vi "AKD Set Drive Enable.vi"(0 "connection ID":refnum<k5>, 11 "error in":errorcluster) -> (4 "TCP Refnum":refnum<k5>, 15 "error out":errorcluster)   [LabVIEW 2019]
uses:
  MODBUS/NI Modbus.llb/MB Ethernet Master Query Write Multiple Registers (poly).vi
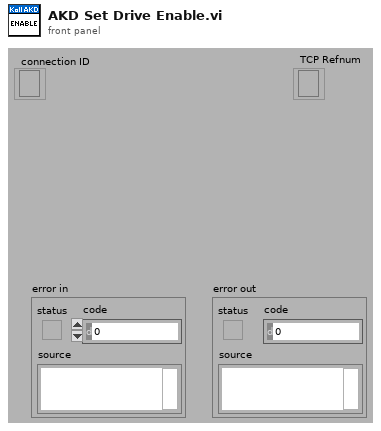
[diagram p1: front panel]
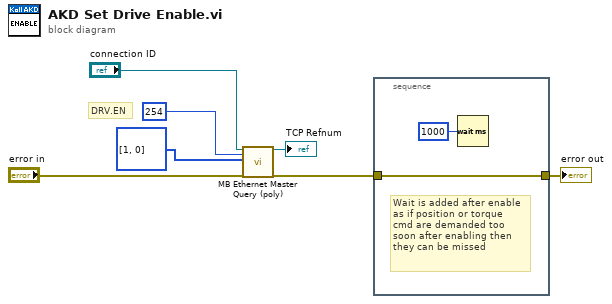
[diagram p0: block diagram]
diagram:
  # "DRV.EN"
  n1 = call-poly "MB Ethernet Master Query (poly).vi"("TCP Connection Refnum in"="connection ID", "Starting Address"=u16 254, "Registers"=u16[] [1, 0], "error in"="error in") -> ("TCP Connection Refnum (dup)"=→"TCP Refnum":refnum<k5>, "error out"=w1:errorcluster)  [unwired: 13 in, 1 out]
  n2 = stacked-sequence {
    tunnel: [w9] -> w2
    tunnel: w1 -> [w9]
    frame #0 {
      # "Wait is added after enable\nas if position or torque \ncmd are demanded too\nsoon after enabling then\nthey can be missed"
      n3 = Wait (ms)(milliseconds to wait=u32 1000) -> ()  [unwired: 1 out]
    }
  }
  "error out" <- w2
